vi "set_modelock_search.vi"(8 "error in (no error)":errorcluster, 10 "modelock search":bool, 11 "LightSourceAN191011Chameleon in":refnum<class "LightSourceAN191011Chameleon.lvclass">) -> (0 "error out":errorcluster, 3 "LightSourceAN191011Chameleon out":refnum<class "LightSourceAN191011Chameleon.lvclass">)   [LabVIEW 2010, in "LightSourceAN191011Chameleon.lvclass"]
uses:
  LightSourceAN191011Chameleon.lvclass
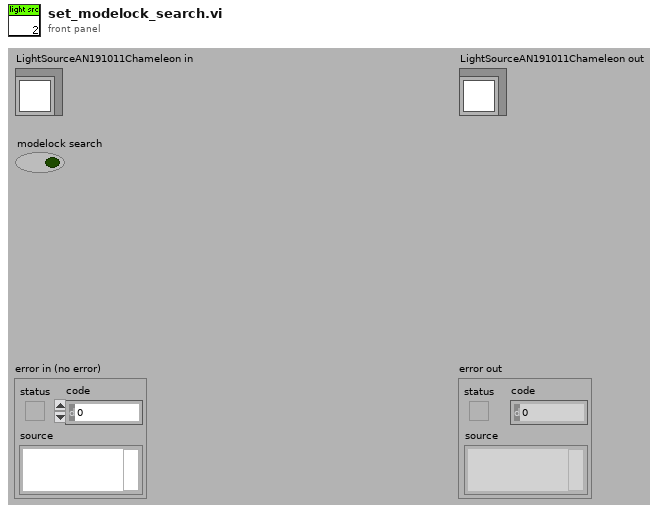
[diagram p1: front panel]
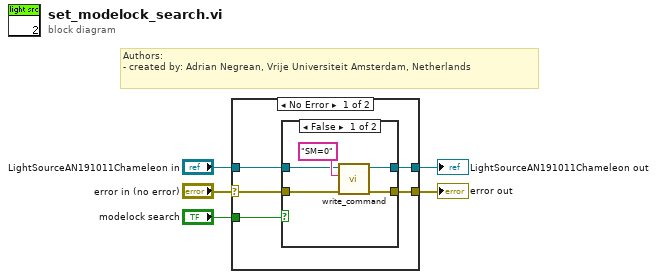
[diagram p0: block diagram]
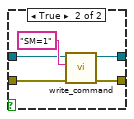
[diagram p2: hidden frame]
diagram:
  # "Authors: \n- created by: Adrian Negrean, Vrije Universiteit Amsterdam, Netherlands"
  n1 = case shown="No Error" "error in (no error)" {
    selector: "error in (no error)" -> [w8 w22]
    tunnel: [w7 w22] -> w4
    tunnel: [w9 w21] -> w2
    tunnel: "LightSourceAN191011Chameleon in" -> [w10 w21]
    tunnel: "modelock search" -> [w6 _]
    frame No Error {
      n2 = case shown="False" w6 {
        tunnel: w10 -> [w14 w19]
        tunnel: [w13 w18] -> w9
        tunnel: w8 -> [w12 w17]
        tunnel: [w11 w16] -> w7
        frame False {
          n3 = call-dynamic "write_command.vi"("error in (no error)"=w12, "string to write"="SM=0", "LightSourceAN191011Chameleon in"=w14) -> ("error out"=w11:errorcluster, "LightSourceAN191011Chameleon out"=w13:refnum<class "LightSourceAN191011Chameleon.lvclass">)  [unwired: 6 in, 1 out]
        }
        frame True {
          n4 = call-dynamic "write_command.vi"("error in (no error)"=w17, "string to write"="SM=1", "LightSourceAN191011Chameleon in"=w19) -> ("error out"=w16:errorcluster, "LightSourceAN191011Chameleon out"=w18:refnum<class "LightSourceAN191011Chameleon.lvclass">)  [unwired: 6 in, 1 out]
        }
      }
    }
    frame Error {
    }
  }
  "error out" <- w4
  "LightSourceAN191011Chameleon out" <- w2
